vi "Add Node Terminals_2014.vi"(6 "Variant in":variant, 7 "Shift Pressed?":bool, 8 "error in (no error)":errorcluster, 10 "QD Combo Box Ref":refnum<vi>, 11 "QD Launch VI Ref":refnum<vi>) -> (0 "error out":errorcluster, 4 "Variant out":variant)   [LabVIEW 2015]
doc: "Add terminal to any bundler, unbundler, merge error, concatinate string, index array, decimate array, interleave array or build array/matrix selecting the node, starting quick drop and hitting Ctl-N. A specific number of terminals can be selected by entering it into the text box or hitting space the same number as terminals that are desired. A single terminal can be removed by hitting Ctl-Shift-N.\n\nNEW: Add/Remove terminals to Property Node. A terminal can be added to a property node by selecting the property node, launching quick drop, and hitting Ctl-N. A specific number of terminals can be added by entering it into the text box or hitting space as many times as desired terminals to be added. A single terminal can be removed by hitting Ctl-Shift-N or multiple terminals removed by entering the number desired to be removed or entering space as many times as terminals to be removed and then hitting Ctl-Shift-N.\n\nDefault Shortcut - [N]"
panel:
  in  "Undo Name":string="Quick Drop Keyboard Shortcut"
  # "Do not change the connector pane of this VI.\n\nSee the block diagram for directions on how to use this template."
  # "Specify the name of the Undo transaction"
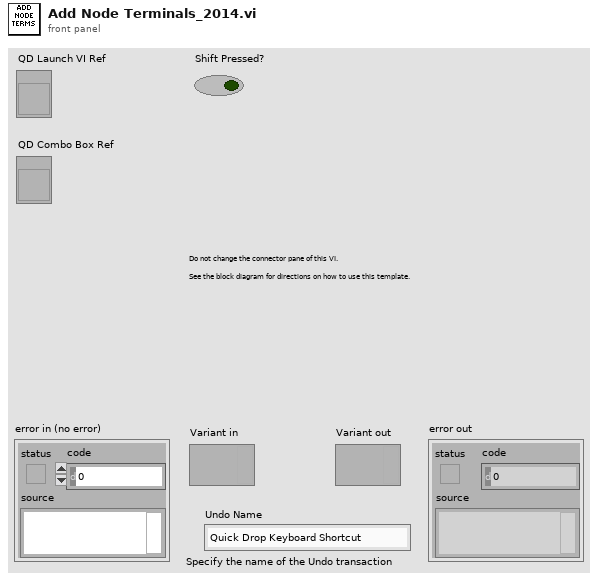
[diagram p1: front panel]
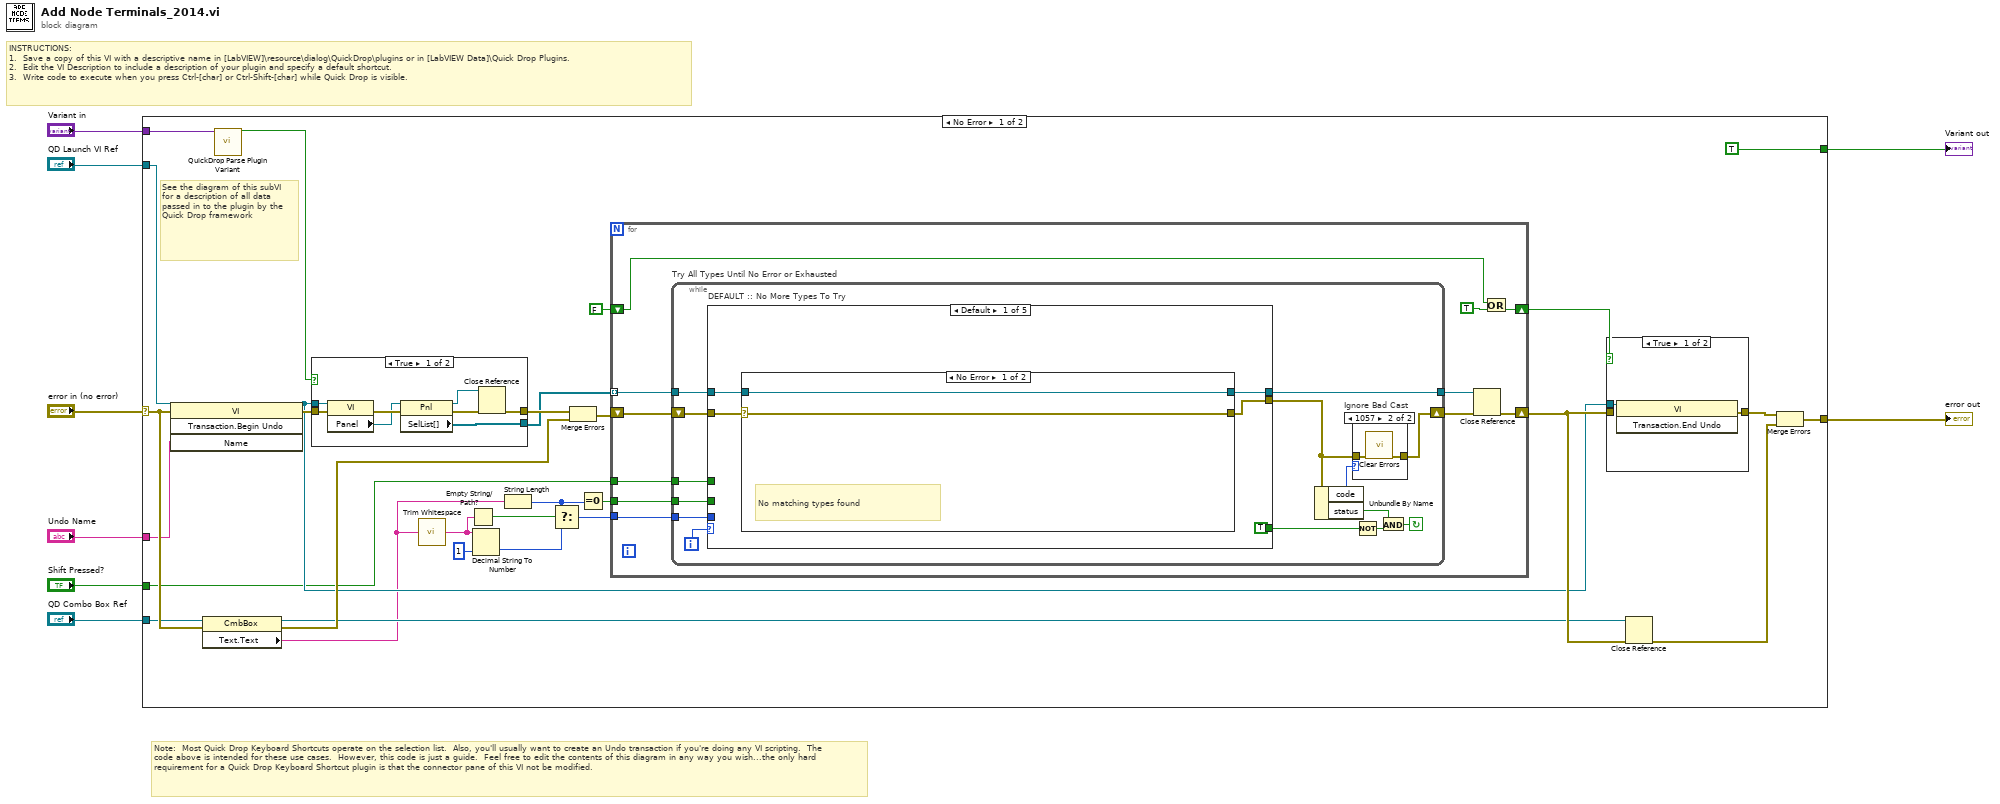
[diagram p0: block diagram]
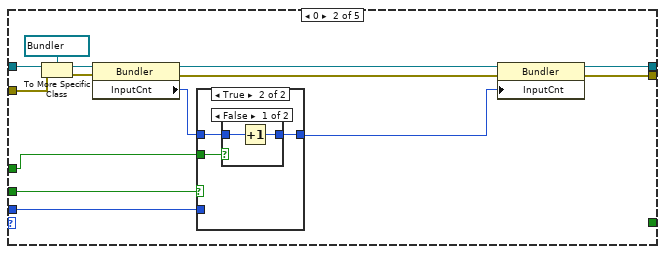
[diagram p4: hidden frame]
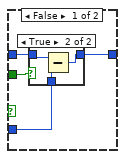
[diagram p5: hidden frame]
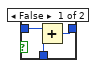
[diagram p6: hidden frame]
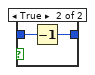
[diagram p7: hidden frame]
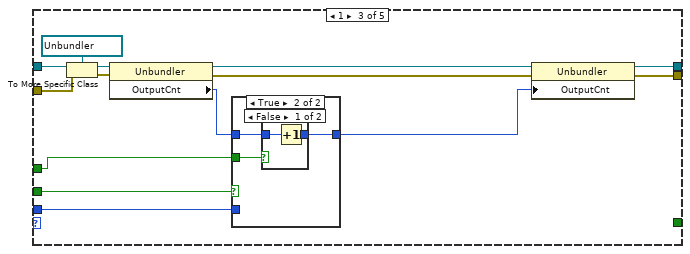
[diagram p8: hidden frame]
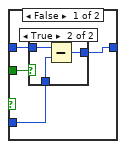
[diagram p9: hidden frame]
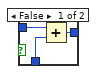
[diagram p10: hidden frame]
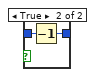
[diagram p11: hidden frame]
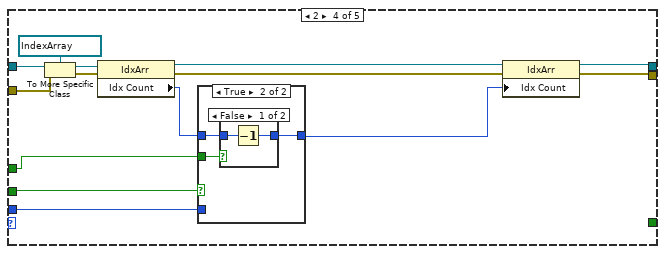
[diagram p12: hidden frame]
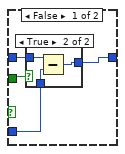
[diagram p13: hidden frame]
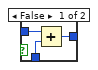
[diagram p14: hidden frame]
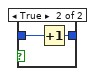
[diagram p15: hidden frame]
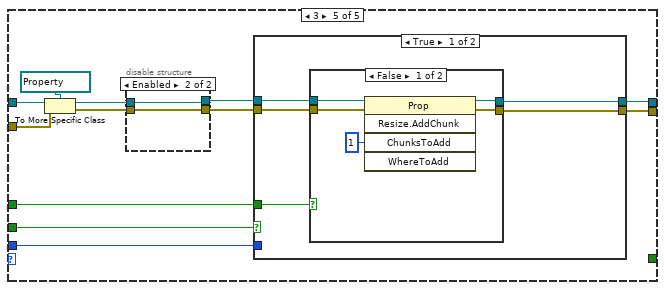
[diagram p16: hidden frame]
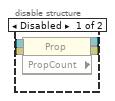
[diagram p17: hidden frame]
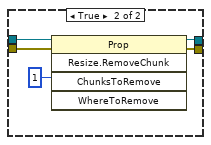
[diagram p18: hidden frame]
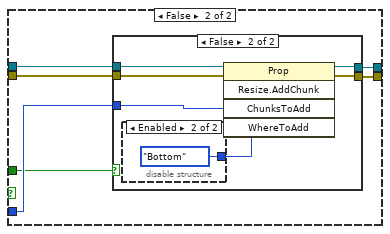
[diagram p19: hidden frame]
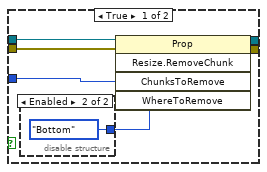
[diagram p20: hidden frame]
diagram:
  # "Note:  Most Quick Drop Keyboard Shortcuts operate on the selection list.  Also, you'll usually want to create an Undo transaction if you're doing any VI scripting.  The code above is intended for these use cases.  However, this code is just a guide.  Feel free to edit the contents of this diagram in any way you wish...the only hard requirement for a Quick Drop Keyboard Shortcut plugin is that the connector pane of this VI not be modified."
  # "INSTRUCTIONS:\n1.  Save a copy of this VI with a descriptive name in [LabVIEW]\\resource\\dialog\\QuickDrop\\plugins or in [LabVIEW Data]\\Quick Drop Plugins.\n2.  Edit the VI Description to include a description of your plugin and specify a default shortcut. \n3.  Write code to execute when you press Ctrl-[char] or Ctrl-Shift-[char] while Quick Drop is visible."
  n1 = case shown="No Error" "error in (no error)" {
    selector: "error in (no error)" -> [w36 w247]
    tunnel: [w23 w247] -> w7
    tunnel: "QD Launch VI Ref" -> [w33 _]
    tunnel: "Shift Pressed?" -> [w10 _]
    tunnel: "QD Combo Box Ref" -> [w25 _]
    tunnel: "Variant in" -> [w34 _]
    tunnel: "Undo Name" -> [w32 _]
    tunnel: [TRUE _] -> w1
    frame No Error {
      # "See the diagram of this subVI for a description of all data passed in to the plugin by the Quick Drop framework"
      n2 = invoke class="VI" method="Transaction.Begin Undo"(reference=w33, error in=w36, "Name"=w32) -> (reference out=w26:refnum<vi>, error out=w29:errorcluster)  [unwired: 1 in, 2 out]
      n3 = property class="CmbBox"(reference=w25, error in=w36) -> (reference out=w24:refnum<vi>, error out=w35:errorcluster, "Text.Text"=w15:string)
      n4 = call <vilib>:"QuickDrop Parse Plugin Variant.vi"("QDKS Variant in"=w34) -> ("QD Launch VI Panel?"=w30:bool)  [unwired: 12 in, 2 out]
      n5 = case shown="True" w30 {
        tunnel: w29 -> [w238 w246]
        tunnel: w26 -> [w237 w245]
        tunnel: [w232 w240] -> w27
        tunnel: [w231 w239] -> w20
        frame True {
          n6 = property class="VI"(reference=w237, error in=w238) -> (error out=w236:errorcluster, "Panel"=w235:refnum<vi>)  [unwired: 1 out]
          n7 = property class="Pnl"(reference=w235, error in=w236) -> (reference out=w233:refnum<vi>, error out=w234:errorcluster, "SelList[]"=w231:refnum<vi>[])
          n8 = Close Reference(reference=w233, error in (no error)=w234) -> (error out=w232:errorcluster)
        }
        frame False {
          n9 = property class="VI"(reference=w245, error in=w246) -> (error out=w244:errorcluster, "Diagram"=w243:refnum<vi>)  [unwired: 1 out]
          n10 = property class="TopLvlDiag"(reference=w243, error in=w244) -> (reference out=w241:refnum<vi>, error out=w242:errorcluster, "SelList[]"=w239:refnum<vi>[])
          n11 = Close Reference(reference=w241, error in (no error)=w242) -> (error out=w240:errorcluster)
        }
      }
      n12 = call <vilib>:"Trim Whitespace.vi"("string"=w15) -> ("trimmed string"=w16:string)  [unwired: 1 in]
      n13 = Empty String/Path?(string/path=w16) -> (empty?=w13:bool)
      n14 = Decimal String To Number(string=w16, default (0L)=1 ("default (0 I32)")) -> (number=w9:i32)  [unwired: 1 in, 1 out]
      n15 = String Length(string=w15) -> (length=w12:i32)
      n16 = Select(t=w12, s=w13, f=w9) -> (s? t:f=w14:i32)
      n17 = Merge Errors(w27, w35) -> (w21:errorcluster)
      n18 = Equal To 0?(x=w12) -> (x = 0?=w11:bool)
      n19 = for {
        shift-right: [w48] -> w37
        shift-left: w21 -> [w39]
        tunnel: w20 -> [w44] mode=indexing
        shift-right: [w46] -> w18
        shift-left: FALSE -> [w47]
        tunnel: w14 -> [w42]
        tunnel: w11 -> [w43]
        tunnel: w10 -> [w38]
        n20 = while "Try All Types Until No Error or Exhausted" {
          tunnel: w44 -> [w62]
          tunnel: [w61] -> w41
          shift-right: [w54] -> w40
          shift-left: w39 -> [w56]
          tunnel: w43 -> [w51]
          tunnel: w42 -> [w50]
          tunnel: w38 -> [w49]
          i -> [w60]
          stop <- w59 continue-if-true
          n21 = case "DEFAULT :: No More Types To Try" shown="Default" w60 {
            tunnel: w56 -> [w67 w88 w119 w150 w179]
            tunnel: w62 -> [w68 w86 w117 w148 w177]
            tunnel: [w69 w79 w109 w141 w170] -> w61
            tunnel: [w66 w81 w111 w143 w169] -> w53
            tunnel: [TRUE _ _ _ _] -> w58
            tunnel: w51 -> [_ w77 w112 w139 w173]
            tunnel: w50 -> [_ w76 w107 w138 w174]
            tunnel: w49 -> [_ w75 w106 w137 w168]
            frame Default {
              n22 = case shown="No Error" w67 {
                selector: w67 -> [w71 w73]
                tunnel: [w72 w74] -> w69
                tunnel: w68 -> [w72 w74]
                tunnel: [w71 w73] -> w66
                frame No Error {
                  # "No matching types found"
                }
                frame Error {
                  # "No matching types found\n\nAllow this non-typecast error to propogate through without modification"
                }
              }
            }
            frame 0 {
              n23 = To More Specific Class(target class=refnum<vi> refnum ("Waveform Chart"), reference=w86, error in=w88) -> (specific class reference=w83:refnum<vi>, error out=w85:errorcluster)
              n24 = property class="Bundler"(reference=w83, error in=w85) -> (reference out=w80:refnum<vi>, error out=w84:errorcluster, "InputCnt"=w82:i32)
              n25 = case shown="True" w77 {
                tunnel: w82 -> [w90 w100]
                tunnel: [w91 w101] -> w78
                tunnel: w76 -> [w92 _]
                tunnel: w75 -> [w89 w99]
                frame False {
                  n26 = case shown="True" w89 {
                    tunnel: w92 -> [w95 w97]
                    tunnel: [w94 w96] -> w91
                    tunnel: w90 -> [w93 w98]
                    frame False {
                      n27 = Add(x=w93, y=w95) -> (x+y=w94:i32)
                    }
                    frame True {
                      n28 = Subtract(x=w98, y=w97) -> (x-y=w96:i32)
                    }
                  }
                }
                frame True {
                  n29 = case shown="False" w99 {
                    tunnel: [w103 w104] -> w101
                    tunnel: w100 -> [w102 w105]
                    frame False {
                      n30 = Increment(x=w102) -> (x+1=w103:i32)
                    }
                    frame True {
                      n31 = Decrement(x=w105) -> (x-1=w104:i32)
                    }
                  }
                }
              }
              n32 = property class="Bundler"(reference=w80, error in=w84, "InputCnt"=w78) -> (reference out=w79:refnum<vi>, error out=w81:errorcluster)
            }
            frame 1 {
              n33 = To More Specific Class(target class=refnum<vi> refnum ("Waveform Chart"), reference=w117, error in=w119) -> (specific class reference=w114:refnum<vi>, error out=w116:errorcluster)
              n34 = property class="Unbundler"(reference=w114, error in=w116) -> (reference out=w110:refnum<vi>, error out=w115:errorcluster, "OutputCnt"=w113:i32)
              n35 = case shown="True" w112 {
                tunnel: w113 -> [w121 w131]
                tunnel: [w122 w132] -> w108
                tunnel: w107 -> [w123 _]
                tunnel: w106 -> [w120 w130]
                frame False {
                  n36 = case shown="True" w120 {
                    tunnel: w123 -> [w126 w128]
                    tunnel: [w125 w127] -> w122
                    tunnel: w121 -> [w124 w129]
                    frame False {
                      n37 = Add(x=w124, y=w126) -> (x+y=w125:i32)
                    }
                    frame True {
                      n38 = Subtract(x=w129, y=w128) -> (x-y=w127:i32)
                    }
                  }
                }
                frame True {
                  n39 = case shown="False" w130 {
                    tunnel: [w134 w135] -> w132
                    tunnel: w131 -> [w133 w136]
                    frame False {
                      n40 = Increment(x=w133) -> (x+1=w134:i32)
                    }
                    frame True {
                      n41 = Decrement(x=w136) -> (x-1=w135:i32)
                    }
                  }
                }
              }
              n42 = property class="Unbundler"(reference=w110, error in=w115, "OutputCnt"=w108) -> (reference out=w109:refnum<vi>, error out=w111:errorcluster)
            }
            frame 2 {
              n43 = To More Specific Class(target class=refnum<vi> refnum ("Waveform Chart"), reference=w148, error in=w150) -> (specific class reference=w145:refnum<vi>, error out=w147:errorcluster)
              n44 = property class="IdxArr"(reference=w145, error in=w147) -> (reference out=w142:refnum<vi>, error out=w146:errorcluster, "Idx Count"=w144:i32)
              n45 = case shown="True" w139 {
                tunnel: w144 -> [w152 w162]
                tunnel: [w153 w163] -> w140
                tunnel: w138 -> [w154 _]
                tunnel: w137 -> [w151 w161]
                frame False {
                  n46 = case shown="True" w151 {
                    tunnel: w154 -> [w157 w159]
                    tunnel: [w156 w158] -> w153
                    tunnel: w152 -> [w155 w160]
                    frame False {
                      n47 = Add(x=w155, y=w157) -> (x+y=w156:i32)
                    }
                    frame True {
                      n48 = Subtract(x=w160, y=w159) -> (x-y=w158:i32)
                    }
                  }
                }
                frame True {
                  n49 = case shown="False" w161 {
                    tunnel: [w164 w167] -> w163
                    tunnel: w162 -> [w165 w166]
                    frame False {
                      n50 = Decrement(x=w165) -> (x-1=w164:i32)
                    }
                    frame True {
                      n51 = Increment(x=w166) -> (x+1=w167:i32)
                    }
                  }
                }
              }
              n52 = property class="IdxArr"(reference=w142, error in=w146, "Idx Count"=w140) -> (reference out=w141:refnum<vi>, error out=w143:errorcluster)
            }
            frame 3 {
              n53 = To More Specific Class(target class=refnum<vi> refnum ("Waveform Chart"), reference=w177, error in=w179) -> (specific class reference=w175:refnum<vi>, error out=w176:errorcluster)
              n54 = disable-structure shown="Enabled" {
                disable-tunnel: w176 -> [w183 w184]
                disable-tunnel: w175 -> [w182 w185]
                disable-tunnel: [w181 w185] -> w172
                disable-tunnel: [w180 w184] -> w171
                frame Disabled {
                  n55 = property class="Prop" props=["PropCount"](reference=w182, error in=w183) -> (reference out=w181:refnum<vi>, error out=w180:errorcluster)  [unwired: 1 out]
                }
                frame Enabled {
                }
              }
              n56 = case shown="True" w173 {
                tunnel: w174 -> [_ w202]
                tunnel: w172 -> [w190 w206]
                tunnel: w171 -> [w189 w205]
                tunnel: [w188 w204] -> w170
                tunnel: [w187 w203] -> w169
                tunnel: w168 -> [w186 w201]
                frame True {
                  n57 = case shown="False" w186 {
                    tunnel: w190 -> [w194 w199]
                    tunnel: w189 -> [w193 w198]
                    tunnel: [w192 w197] -> w188
                    tunnel: [w191 w196] -> w187
                    frame False {
                      n58 = invoke class="Prop" method="Resize.AddChunk"(reference=w194, error in=w193, "ChunksToAdd"=u8 1 ("Chunks To Add")) -> (reference out=w192:refnum<vi>, error out=w191:errorcluster)  [unwired: 2 in, 3 out]
                    }
                    frame True {
                      n59 = invoke class="Prop" method="Resize.RemoveChunk"(reference=w199, error in=w198, "ChunksToRemove"=u8 1 ("Chunks To Add")) -> (reference out=w197:refnum<vi>, error out=w196:errorcluster)  [unwired: 2 in, 3 out]
                    }
                  }
                }
                frame False {
                  n60 = case shown="False" w201 {
                    tunnel: w206 -> [w212 w222]
                    tunnel: w205 -> [w211 w221]
                    tunnel: [w210 w220] -> w204
                    tunnel: [w209 w219] -> w203
                    tunnel: w202 -> [w207 w217]
                    frame True {
                      n61 = disable-structure shown="Enabled" {
                        disable-tunnel: [w213 enum8{"Bottom", "Top"}."Bottom" ("Where To Remove")] -> w208
                        frame Disabled {
                          n62 = case shown="False" {
                            selector: _ -> [_ _]
                            tunnel: [enum8{"Bottom", "Top"}."Top" ("Where To Remove") enum8{"Bottom", "Top"}."Bottom" ("Where To Remove")] -> w213
                            frame True {
                            }
                            frame False {
                            }
                          }
                        }
                        frame Enabled {
                        }
                      }
                      n63 = invoke class="Prop" method="Resize.RemoveChunk"(reference=w212, error in=w211, "ChunksToRemove"=w207, "WhereToRemove"=w208) -> (reference out=w210:refnum<vi>, error out=w209:errorcluster)  [unwired: 1 in, 3 out]
                    }
                    frame False {
                      n64 = disable-structure shown="Enabled" {
                        disable-tunnel: [w223 enum8{"Bottom", "Top"}."Bottom" ("Where To Remove")] -> w218
                        frame Disabled {
                          n65 = case shown="False" {
                            selector: _ -> [_ _]
                            tunnel: [enum8{"Bottom", "Top"}."Top" ("Where To Remove") enum8{"Bottom", "Top"}."Bottom" ("Where To Remove")] -> w223
                            frame True {
                            }
                            frame False {
                            }
                          }
                        }
                        frame Enabled {
                        }
                      }
                      n66 = invoke class="Prop" method="Resize.AddChunk"(reference=w222, error in=w221, "ChunksToAdd"=w217, "WhereToAdd"=w218) -> (reference out=w220:refnum<vi>, error out=w219:errorcluster)  [unwired: 1 in, 3 out]
                    }
                  }
                }
              }
            }
          }
          n67 = Unbundle By Name(w53) -> ("code"=w52:i32, "status"=w55:bool)
          n68 = case "Ignore Bad Cast" shown="1057" w52 {
            tunnel: [w63 w65] -> w54
            tunnel: w53 -> [w63 w64]
            frame Default {
            }
            frame 1057 {
              n69 = call <vilib>:"Clear Errors.vi"("error in (no error)"=w64) -> ("error out"=w65:errorcluster)  [unwired: 5 in, 1 out]
            }
          }
          n70 = Not(x=w58) -> (.not. x?=w57:bool)
          n71 = And(x=w55, y=w57) -> (x .and. y?=w59:bool)
        }
        n72 = Close Reference(reference=w41, error in (no error)=w40) -> (error out=w48:errorcluster)
        n73 = Or(x=w47, y=TRUE ("x")) -> (x .or. y?=w46:bool)
      }
      n74 = case shown="True" w18 {
        tunnel: w26 -> [w227 w229]
        tunnel: [w228 w230] -> w28
        tunnel: w37 -> [_ _]
        frame True {
          n75 = invoke class="VI" method="Transaction.End Undo"(reference=w227) -> (error out=w228:errorcluster)  [unwired: 2 in, 2 out]
        }
        frame False {
          n76 = invoke class="VI" method="Transaction.Fail"(reference=w229) -> (error out=w230:errorcluster)  [unwired: 2 in, 2 out]
        }
      }
      n77 = Close Reference(reference=w24, error in (no error)=w37) -> (error out=w22:errorcluster)
      n78 = Merge Errors(w28, w22) -> (w23:errorcluster)
    }
    frame Error {
    }
  }
  "error out" <- w7
  "Variant out" <- w1
